vi "main.vi"   [LabVIEW 2010, in "Poller_Main.lvclass"]
uses:
  Poller_Main.lvclass
  protocols/protocol_Generic/Protocol_Generic.lvclass
  protocols/protocol_MoveToSetpoint/Protocol_MoveToSetpoint.lvclass
  protocols/protocol_Logging/Protocol_Logging.lvclass
types:
  T1 = cluster{"Protocol_MoveToSetpoint.lvclass":refnum<class "Protocol_MoveToSetpoint.lvclass">, "Protocol_Logging.lvclass":refnum<class "Protocol_Logging.lvclass">, "Protocol_Generic.lvclass":refnum<class "Protocol_Generic.lvclass">}
  T2 = cluster{"Axis Information":cluster{"Device ID":i32, "Device Name":string, "Device Type":i32}[], "Axis Selector":i32[], "Control Modes out":u16[], "error out":errorcluster, "Channel Data":cluster{"Name":string, "Type":i32, "SI Full Scale":dbl, "Full Scale":dbl, "Units String":string, "Display Format":string, "Gauge Length":dbl}[][]}
  T3 = cluster{"Name":string, "Type":i32, "SI Full Scale":dbl, "Full Scale":dbl, "Units String":string, "Display Format":string, "Gauge Length":dbl}[][]
  T4 = cluster{"Device ID":i32, "Device Name":string, "Device Type":i32}[]
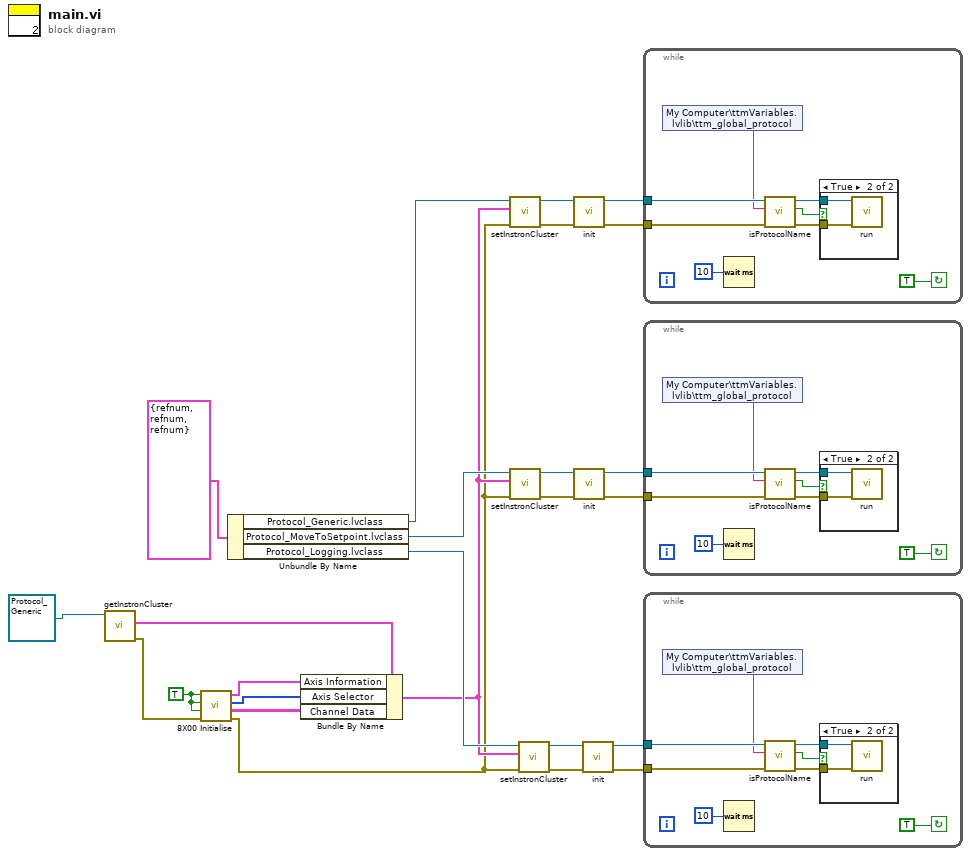
[diagram p0: block diagram]
diagram:
  w25 = TRUE ("Create Console? (T)")
  n1 = call-dynamic "getInstronCluster.vi"("Protocol_Generic in"=refnum<class "Protocol_Generic.lvclass"> refnum ("Protocol_Generic.lvclass")) -> ("error out"=w19:errorcluster, "InstronCluster"=w23:T2)  [unwired: 8 in, 1 out]
  n2 = call "8X00 Initialise.vi"("error in (no error)"=w19, "Reset?"=w25, "Create DVM? (T)"=w25, "Create Console? (T)"=w25) -> ("error out"=w1:errorcluster, "Channel Data"=w20:T3, "Axis Selector"=w21:i32[], "Axis Information"=w22:T4)
  n3 = Unbundle By Name(T1 {"Protocol_MoveToSetpoint.lvclass"=refnum, "Protocol_Logging.lvclass"=refnum, "Protocol_Generic.lvclass"=refnum}) -> ("Protocol_Generic.lvclass"=w3:refnum<class "Protocol_Generic.lvclass">, "Protocol_MoveToSetpoint.lvclass"=w13:refnum<class "Protocol_MoveToSetpoint.lvclass">, "Protocol_Logging.lvclass"=w10:refnum<class "Protocol_Logging.lvclass">)
  n4 = Bundle By Name(cluster=w23, "Axis Information"=w22, "Axis Selector"=w21, "Channel Data"=w20) -> (w2:T2)
  n5 = call-dynamic "setInstronCluster.vi"("error in (no error)"=w1, "InstronCluster"=w2, "Protocol_Generic in"=w3) -> ("error out"=w6:errorcluster, "Protocol_Generic out"=w7:refnum<class "Protocol_Generic.lvclass">)  [unwired: 7 in]
  n6 = call-dynamic "setInstronCluster.vi"("error in (no error)"=w1, "InstronCluster"=w2, "Protocol_Generic in"=w13) -> ("error out"=w17:errorcluster, "Protocol_Generic out"=w18:refnum<class "Protocol_MoveToSetpoint.lvclass">)  [unwired: 7 in]
  n7 = call-dynamic "setInstronCluster.vi"("error in (no error)"=w1, "InstronCluster"=w2, "Protocol_Generic in"=w10) -> ("error out"=w12:errorcluster, "Protocol_Generic out"=w11:refnum<class "Protocol_Logging.lvclass">)  [unwired: 7 in]
  n8 = call-dynamic "init.vi"("error in (no error)"=w6, "Protocol_Generic in"=w7) -> ("error out"=w4:errorcluster, "Protocol_Generic out"=w5:refnum<class "Protocol_Generic.lvclass">)  [unwired: 8 in]
  n9 = call-dynamic "init.vi"("error in (no error)"=w17, "Protocol_MoveToSetpoint in"=w18) -> ("error out"=w15:errorcluster, "Protocol_MoveToSetpoint out"=w16:refnum<class "Protocol_MoveToSetpoint.lvclass">)  [unwired: 8 in]
  n10 = call-dynamic "init.vi"("error in (no error)"=w12, "Protocol_Logging in"=w11) -> ("error out"=w8:errorcluster, "Protocol_Logging out"=w9:refnum<class "Protocol_Logging.lvclass">)  [unwired: 8 in]
  n11 = while {
    tunnel: w5 -> [w33]
    tunnel: w4 -> [w32]
    stop <- TRUE continue-if-true
    n12 = shared-variable "My Computer\\ttmVariables.lvlib\\ttm_global_protocol"() -> (w31:string)  [unwired: 1 in, 1 out]
    n13 = Wait (ms)(milliseconds to wait=u32 10) -> ()  [unwired: 1 out]
    n14 = call-dynamic "isProtocolName.vi"("error in (no error)"=w32, "name"=w31, "Protocol_Generic in"=w33) -> ("error out"=w28:errorcluster, "isName"=w30:bool, "Protocol_Generic out"=w29:refnum<class "Protocol_Generic.lvclass">)  [unwired: 6 in]
    n15 = case shown="True" w30 {
      tunnel: w29 -> [_ w35]
      tunnel: w28 -> [_ w34]
      frame False {
      }
      frame True {
        n16 = call-dynamic "run.vi"("error in (no error)"=w34, "Protocol_Generic in"=w35) -> ()  [unwired: 8 in, 2 out]
      }
    }
  }
  n17 = while {
    tunnel: w16 -> [w43]
    tunnel: w15 -> [w42]
    stop <- TRUE continue-if-true
    n18 = shared-variable "My Computer\\ttmVariables.lvlib\\ttm_global_protocol"() -> (w41:string)  [unwired: 1 in, 1 out]
    n19 = Wait (ms)(milliseconds to wait=u32 10) -> ()  [unwired: 1 out]
    n20 = call-dynamic "isProtocolName.vi"("error in (no error)"=w42, "name"=w41, "Protocol_Generic in"=w43) -> ("error out"=w38:errorcluster, "isName"=w40:bool, "Protocol_Generic out"=w39:refnum<class "Protocol_MoveToSetpoint.lvclass">)  [unwired: 6 in]
    n21 = case shown="True" w40 {
      tunnel: w39 -> [_ w45]
      tunnel: w38 -> [_ w44]
      frame False {
      }
      frame True {
        n22 = call-dynamic "run.vi"("error in (no error)"=w44, "Protocol_MoveToSetpoint in"=w45) -> ()  [unwired: 8 in, 2 out]
      }
    }
  }
  n23 = while {
    tunnel: w9 -> [w53]
    tunnel: w8 -> [w52]
    stop <- TRUE continue-if-true
    n24 = shared-variable "My Computer\\ttmVariables.lvlib\\ttm_global_protocol"() -> (w51:string)  [unwired: 1 in, 1 out]
    n25 = Wait (ms)(milliseconds to wait=u32 10) -> ()  [unwired: 1 out]
    n26 = call-dynamic "isProtocolName.vi"("error in (no error)"=w52, "name"=w51, "Protocol_Generic in"=w53) -> ("error out"=w48:errorcluster, "isName"=w50:bool, "Protocol_Generic out"=w49:refnum<class "Protocol_Logging.lvclass">)  [unwired: 6 in]
    n27 = case shown="True" w50 {
      tunnel: w49 -> [_ w55]
      tunnel: w48 -> [_ w54]
      frame False {
      }
      frame True {
        n28 = call-dynamic "run.vi"("error in (no error)"=w54, "Protocol_Logging in"=w55) -> ()  [unwired: 8 in, 2 out]
      }
    }
  }
